vi "verify generic related parameters.vi"(8 "error in (no error)":errorcluster, 11 "Simulated_CCD_Camera in":refnum<class "Simulated_CCD_Camera.lvclass">) -> (0 "error out":errorcluster, 3 "Simulated_CCD_Camera out":refnum<class "Simulated_CCD_Camera.lvclass">)   [LabVIEW 2018, in "Simulated_CCD_Camera.lvclass"]
doc: "Verify the related parameters of the camera\n\nThere are some parameters of the camera operation mode that depend on the value provided for another parameter. This function verifies if these parameters are in agreement."
uses:
  Simulated_CCD_Camera.lvclass
  Simulated_CCD_Camera.lvclass/Simulated_CCD_Camera.ctl
  <vilib>/ErrorRing/Error Ring.xnode
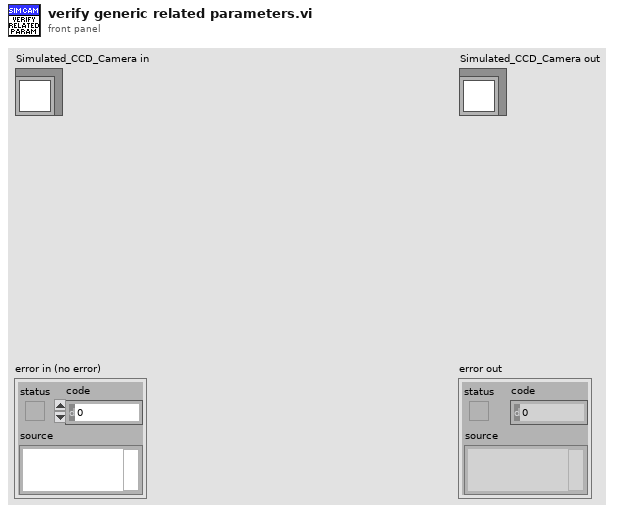
[diagram p1: front panel]
types:
  T1 = cluster{"PREAMP":u16, "READOUT_RATE":u16, "EM_GAIN":u16, "VERTICAL_SHIFT_SPEED":u16, "READ_MODE":u16, "FRAME_TRANSFER":bool, "VERTICAL_CLOCK_VOLTAGE":u16, "ACQUISITION_MODE":u16, "AD_CHANNEL":u16, "EM_MODE":u16, "SHUTTER_TTL":u16, "SHUTTER_OPENING_TIME":u16, "SHUTTER_CLOSING_TIME":u16, "SHUTTER_MODE":u16, "TRIGGER_MODE":u16, "VBIN":u16, "INITIAL_LINE":u16, "INITIAL_COLUMN":u16, "FINAL_LINE":u16, "FINAL_COLUMN":u16, "HBIN":u16}
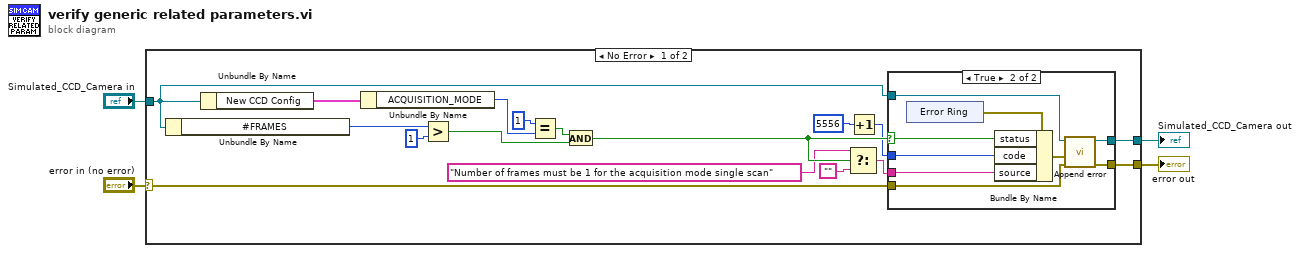
[diagram p0: block diagram]
diagram:
  n1 = case shown="No Error" "error in (no error)" {
    selector: "error in (no error)" -> [w9 w35]
    tunnel: [w8 w35] -> w3
    tunnel: [w10 w34] -> w1
    tunnel: "Simulated_CCD_Camera in" -> [w7 w34]
    frame No Error {
      n2 = Unbundle By Name(w7) -> ("#FRAMES"=w20:u32)
      n3 = Unbundle By Name(w7) -> ("New CCD Config"=w11:T1)
      n4 = Unbundle By Name(w11) -> ("ACQUISITION_MODE"=w21:u16)
      n5 = Greater?(x=w20, y=1) -> (0:w18:bool)
      n6 = Equal?(x=u16 1, y=w21) -> (x = y?=w17:bool)
      n7 = And(x=w17, y=w18) -> (x .and. y?=w16:bool)
      n8 = Select(t="Number of frames must be 1 for the acquisition mode single scan", s=w16, f="") -> (s? t:f=w13:string)
      n9 = Increment(x=5556) -> (x+1=w6:i32)
      n10 = case shown="True" w16 {
        selector: w16 -> [_ w32]
        tunnel: w13 -> [_ w31]
        tunnel: [w23 w28] -> w10
        tunnel: w7 -> [w23 w27]
        tunnel: w9 -> [w22 w26]
        tunnel: [w22 w25] -> w8
        tunnel: w6 -> [_ w24]
        frame False {
        }
        frame True {
          n11 = xnode "Error Ring"() -> ("error out"=w30:errorcluster)
          n12 = Bundle By Name(cluster=w30, "status"=w32, "code"=w24, "source"=w31) -> (w29:errorcluster)
          n13 = call "Append error.vi"("error in (no error)"=w26, "error"=w29, "Simulated_CCD_Camera in"=w27) -> ("error out"=w25:errorcluster, "Simulated_CCD_Camera out"=w28:refnum<class "Simulated_CCD_Camera.lvclass">)  [unwired: 7 in]
        }
      }
    }
    frame Error {
    }
  }
  "error out" <- w3
  "Simulated_CCD_Camera out" <- w1
